vi "WaitNotification.vi"(8 "error in (no error)":errorcluster, 9 "timeout in ms (1000)":i32=1000, 10 "notifier":refnum<notifier>, 11 "ByRefClass in":refnum<class "ClassByRef.lvclass">) -> (0 "error out":errorcluster, 3 "ByRefClass out":refnum<class "ClassByRef.lvclass">)   [LabVIEW 2021, in "ClassUtilities.lvlib" / "ClassByRef.lvclass"]
uses:
  ClassByRef.lvclass
  ClassByRef.lvclass/ClassByRef.ctl
  GetNotifier.vi
  GetNotifier.vi/815770e3-f244-4544-877a-43bf45f14863.vi
  GetRef.vi
  <vilib>/Utility/error.llb/Error Cluster From Error Code.vi
  <vilib>/ErrorRing/Error Ring.xnode
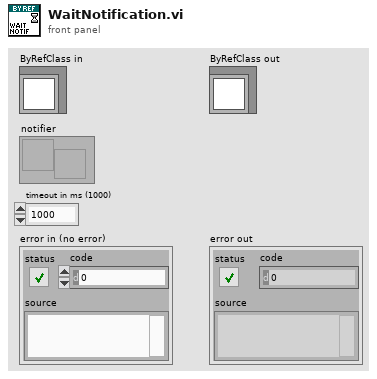
[diagram p1: front panel]
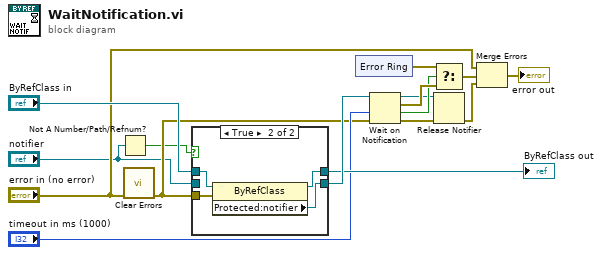
[diagram p0: block diagram]
diagram:
  n1 = Not A Number/Path/Refnum?(number/path/refnum="notifier") -> (NaN/Path/Refnum?=w2:bool)
  n2 = call <vilib>:"Clear Errors.vi"("error in (no error)"="error in (no error)") -> ("error out"=w3:errorcluster)  [unwired: 5 in, 1 out]
  n3 = case shown="True" w2 {
    tunnel: [w18 w22] -> w16
    tunnel: [w17 w21] -> w15
    tunnel: "ByRefClass in" -> [w17 w20]
    tunnel: w3 -> [_ w19]
    tunnel: "notifier" -> [w18 _]
    frame False {
    }
    frame True {
      n4 = property class="ByRefClass"(reference=w20, error in=w19) -> (reference out=w21:refnum<class "ClassByRef.lvclass">, "Protected:notifier"=w22:refnum<notifier>)  [unwired: 1 out]
    }
  }
  "ByRefClass out" <- w15
  n5 = xnode "Error Ring"() -> ("error out"=w13:errorcluster)
  n6 = Wait on Notification(notifier=w16, timeout in ms (-1)="timeout in ms (1000)", error in (no error)=w3) -> (notifier out=w6:refnum<notifier>, notification=w11:errorcluster, timed out?=w10:bool, error out=w8:errorcluster)  [unwired: 1 in]
  n7 = Select(t=w13, s=w10, f=w11) -> (s? t:f=w12:errorcluster)
  n8 = Release Notifier(notifier=w6, error in (no error)=w8) -> (error out=w9:errorcluster)  [unwired: 1 in, 2 out]
  n9 = Merge Errors("error in (no error)", w12, w9) -> (→"error out":errorcluster)
